vi "CU_train_kNN.vi"(6 "DataTypes":T1, 8 "error in (no error)":errorcluster, 9 "Indices":i8[](array[numeric]), 10 "k value":i32, 11 "ClassifierClass in":refnum<class "ClassifierClass.lvclass">) -> (0 "error out":errorcluster, 2 "Classifier Session out":T2, 3 "ClassifierClass out":refnum<class "ClassifierClass.lvclass">)   [LabVIEW 2016, in "Classifier.lvlib" / "ClassifierClass.lvclass"]
uses:
  ClassifierClass.lvclass
  <vilib>/vision/Classification.llb/IMAQ Classifier Session.ctl
  CU_DataTypes.ctl
  <vilib>/vision/Classification.llb/IMAQ Classifier Nearest Neighbor options.ctl
  ClassifierClass.lvclass/ClassifierClass.ctl
  <vilib>/vision/NI_Vision_Development_Module.lvlib
  Classifier.lvlib
panel:
  # "This VI is a part of BCI Design library, http://www.ru-bci.org \nCopyright © 2020, Sotnikov Peter, All rights reserved. License: GNU GPLv3"
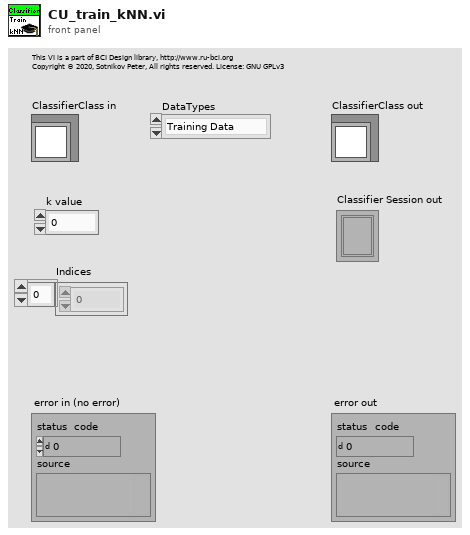
[diagram p1: front panel]
types:
  T1 = typedef "Classifier.lvlib/CU_DataTypes.ctl" = enum16{"Training Data", "Test Data", "Training Data (cross-check)", "Test Data (cross-check)"}
  T2 = typedef "IMAQ Classifier Session.ctl" = refnum<k1>
  T3 = typedef "IMAQ Classifier Nearest Neighbor options.ctl" = cluster{"Method":i32, "Metric":i32, "k":i32}
  T4 = typedef "XML_EEG_Features.lvlib/XML_FF_Trial.ctl" = cluster{"ClassLabel":string, "FeatureVector":dbl[]}
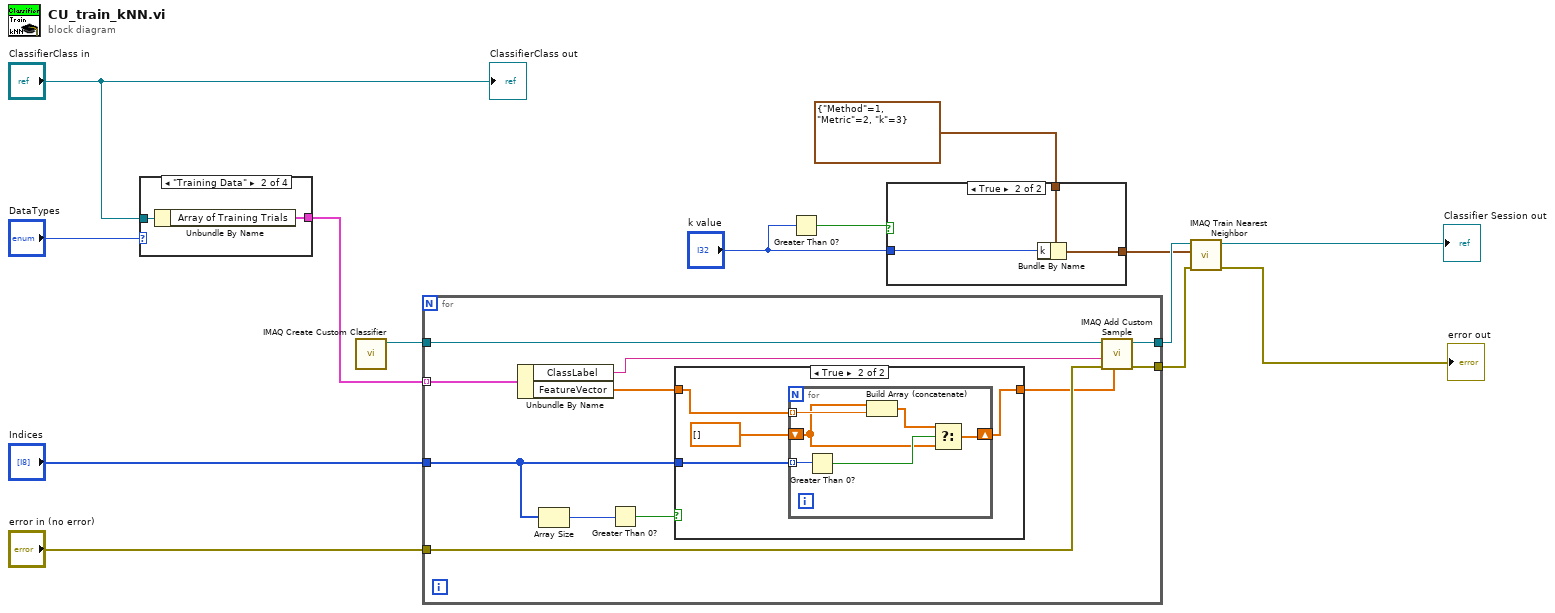
[diagram p0: block diagram]
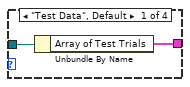
[diagram p2: hidden frame]
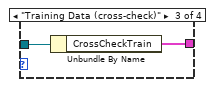
[diagram p3: hidden frame]
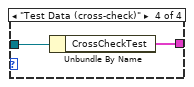
[diagram p4: hidden frame]
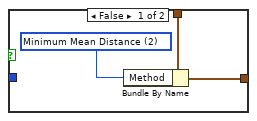
[diagram p5: hidden frame]
diagram:
  n1 = case shown="\"Training Data\"" "DataTypes" {
    tunnel: [w16 w18 w20 w22] -> w1
    tunnel: "ClassifierClass in" -> [w15 w17 w19 w21]
    frame "Test Data", Default {
      n2 = Unbundle By Name(w15) -> ("Array of Test Trials"=w16:T4[])
    }
    frame "Training Data" {
      n3 = Unbundle By Name(w17) -> ("Array of Training Trials"=w18:T4[])
    }
    frame "Training Data (cross-check)" {
      n4 = Unbundle By Name(w19) -> ("CrossCheckTrain"=w20:T4[])
    }
    frame "Test Data (cross-check)" {
      n5 = Unbundle By Name(w21) -> ("CrossCheckTest"=w22:T4[])
    }
  }
  n6 = call "IMAQ Create Custom Classifier"() -> ("Classifier Session"=w9:T2)  [unwired: 10 in, 1 out]
  n7 = for {
    tunnel: w9 -> [w33]
    tunnel: "error in (no error)" -> [w31]
    tunnel: "Indices" -> [w27]
    tunnel: [w26] -> w11
    tunnel: [w25] -> w10
    tunnel: w1 -> [w23] mode=indexing
    n8 = Unbundle By Name(w23) -> ("ClassLabel"=w32:string, "FeatureVector"=w28:dbl[])
    n9 = Array Size(array=w27) -> (size(s)=w30:i32)
    n10 = Greater Than 0?(x=w30) -> (x > 0?=w29:bool)
    n11 = case shown="True" w29 {
      tunnel: w28 -> [w34 w38]
      tunnel: [w34 w35] -> w24
      tunnel: w27 -> [_ w37]
      frame False {
      }
      frame True {
        n12 = for {
          tunnel: w38 -> [w41] mode=indexing
          tunnel: w37 -> [w44] mode=indexing
          shift-right: [w43] -> w35
          shift-left: dbl[] [] -> [w39]
          n13 = Greater Than 0?(x=w44) -> (x > 0?=w42:bool)
          n14 = Build Array (concatenate)(w39, w41) -> (w40:dbl[])
          n15 = Select(t=w40, s=w42, f=w39) -> (s? t:f=w43:dbl[])
        }
      }
    }
    n16 = call "IMAQ Add Custom Sample"("Feature Vector"=w24, "error in (no error)"=w31, "Class"=w32, "Classifier Session"=w33) -> ("error out"=w26:errorcluster, "Classifier Session (dup)"=w25:T2)  [unwired: 6 in]
  }
  n17 = Greater Than 0?(x="k value") -> (x > 0?=w4:bool)
  n18 = case shown="True" w4 {
    tunnel: "k value" -> [_ w50]
    tunnel: T3 {"Method"=1, "Metric"=2, "k"=3} ("Nearest Neighbor Options") -> [w47 w49]
    tunnel: [w46 w48] -> w6
    frame False {
      w45 = 2 items=["Nearest Neighbor", "K Nearest Neighbor", "Minimum Mean Distance"] ("Method")
      n19 = Bundle By Name(cluster=w47, "Method"=w45) -> (w46:T3)
    }
    frame True {
      n20 = Bundle By Name(cluster=w49, "k"=w50) -> (w48:T3)
    }
  }
  n21 = call "IMAQ Train Nearest Neighbor"("error in (no error)"=w11, "Nearest Neighbor Options"=w6, "Classifier Session"=w10) -> ("error out"=→"error out":errorcluster, "Classifier Session (dup)"=→"Classifier Session out":T2)  [unwired: 5 in, 2 out]
  "ClassifierClass out" <- "ClassifierClass in"
